vi "Translate.vi"(0 "reference":refnum<class "AbstractEdge.lvclass">, 1 "dx":dbl format="%.2f", 2 "dy":dbl format="%.2f", 3 "StartEndNode":refnum<class "AbstractNode.lvclass">, 5 "error in (no error)":errorcluster) -> (14 "reference out":refnum<class "AbstractEdge.lvclass">, 19 "error out":errorcluster)   [LabVIEW 2020, in "AbstractEdge.lvclass"]
doc: "Translate edge connection point"
uses:
  <resource>/Framework/Providers/Open_GDS/UML/AbstractEdge_class/AbstractEdge.lvclass
  <resource>/Framework/Providers/Open_GDS/UML/AbstractNode_class/AbstractNode.lvclass
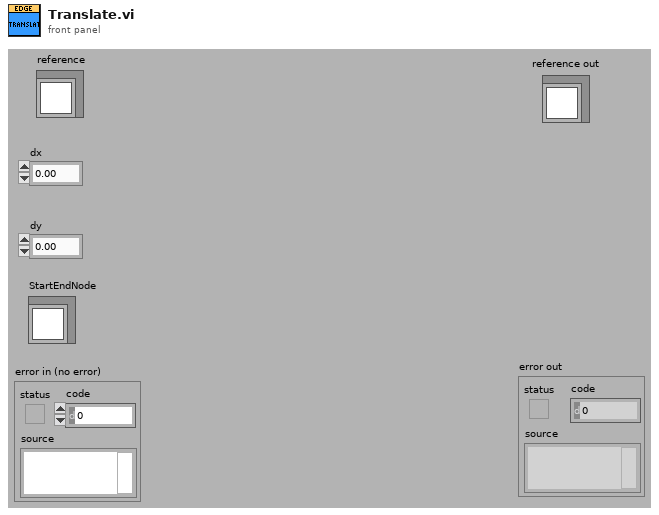
[diagram p1: front panel]
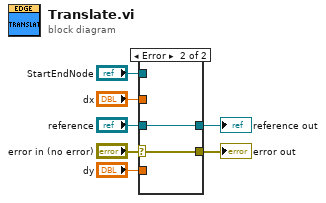
[diagram p0: block diagram]
diagram:
  n1 = case shown="Error" "error in (no error)" {
    selector: "error in (no error)" -> [w8 w10]
    tunnel: "reference" -> [w9 w11]
    tunnel: [w8 w10] -> w6
    tunnel: [w9 w11] -> w5
    tunnel: "dx" -> [_ _]
    tunnel: "dy" -> [_ _]
    tunnel: "StartEndNode" -> [_ _]
    frame No Error {
    }
    frame Error {
    }
  }
  "reference out" <- w5
  "error out" <- w6
